vi "humidity_conversions.vi"() -> ()   [LabVIEW 2026]
panel:
  out "RH SIM":dbl
  out "Sim RH":dbl(graph)
  out "T(C) SIM":dbl
  out "Td SIM":dbl
  out "Sim T(C)":dynamicdata(graph)
  out "Sim Td":dynamicdata(graph)
  in  "stop":bool
  in  "TRUE = RH over water\nFALSE = RH over ice":bool
  out "K":dbl
  in  "T (C)":dbl
  out "Td - out":dbl
  in  "RH - inp":dbl
  # "CONVERTS RH & TEMP TO DEW POINT"
  # "CONVERTS TEMP & DEW POINT TO RH"
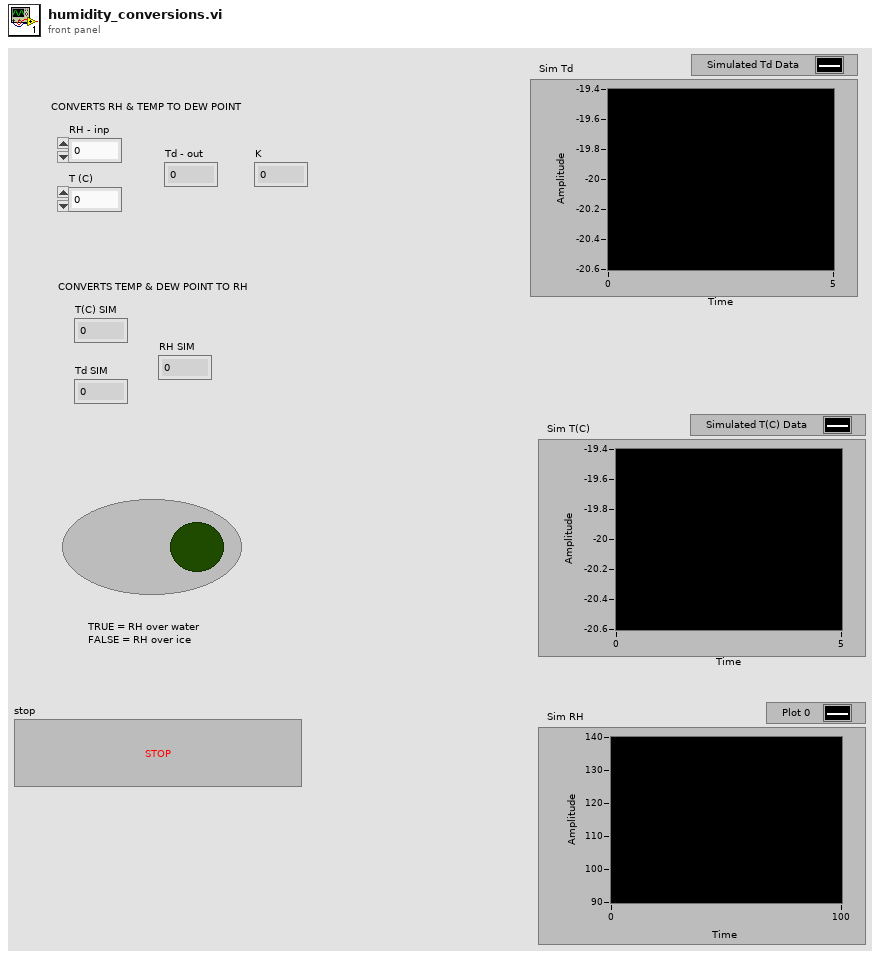
[diagram p1: front panel]
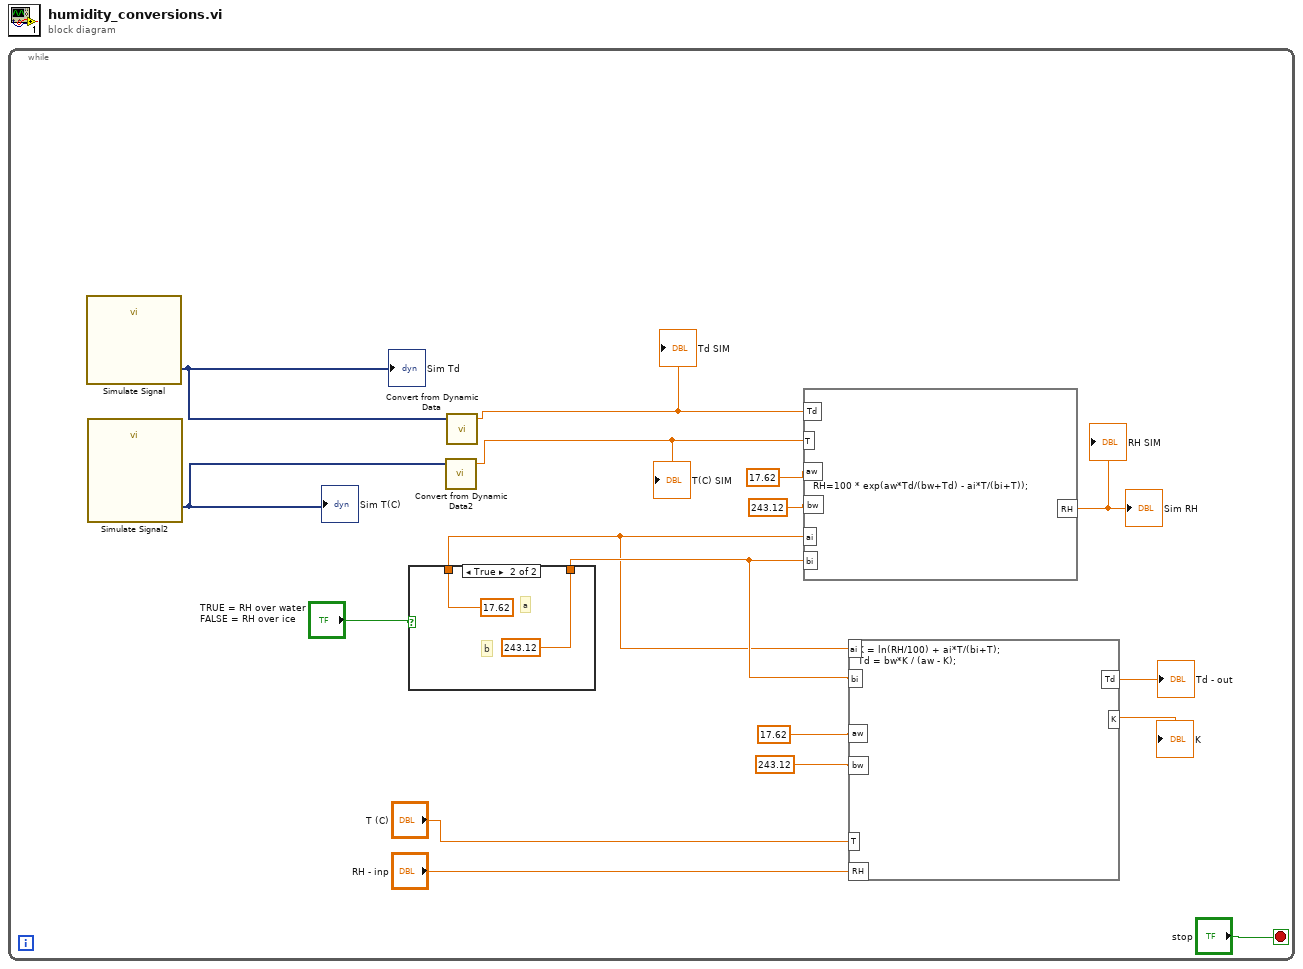
[diagram p0: block diagram]
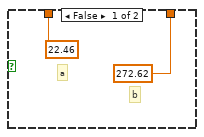
[diagram p2: hidden frame]
diagram:
  n1 = while {
    stop <- "stop" stop-if-true
    n2 = call "Simulate Signal"() -> ("Simulated Td Data"=w5:dynamicdata)  [unwired: 14 in, 1 out]
    "Sim Td" <- w5
    n3 = call "Simulate Signal2"() -> ("Simulated T(C) Data"=w3:dynamicdata)  [unwired: 14 in, 1 out]
    "Sim T(C)" <- w3
    n4 = case shown="True" "TRUE = RH over water\nFALSE = RH over ice" {
      tunnel: [22.46 ("input variable") 17.62 ("input variable")] -> w11
      tunnel: [272.62 ("input variable") 243.12 ("input variable")] -> w14
      frame False {
        # "b"
        # "a"
      }
      frame True {
        # "b"
        # "a"
      }
    }
    n5 = call "Convert from Dynamic Data2"("Dynamic Data Type"=w3) -> ("Scalar"=w2:dbl)  [unwired: 3 in]
    "T(C) SIM" <- w2
    n6 = call "Convert from Dynamic Data"("Dynamic Data Type"=w5) -> ("Scalar"=w4:dbl)  [unwired: 3 in]
    "Td SIM" <- w4
    n7 = formula code="RH=100 * exp(aw*Td/(bw+Td) - ai*T/(bi+T));"("Td"=w4, "T"=w2, "ai"=w11, "bi"=w14, "aw"=17.62 ("input variable"), "bw"=243.12 ("input variable")) -> ("RH"=→"Sim RH" →"RH SIM":dbl)
    n8 = formula code="K = ln(RH/100) + ai*T/(bi+T);\nTd = bw*K / (aw - K);"("RH"="RH - inp", "ai"=w11, "bi"=w14, "T"="T (C)", "aw"=17.62 ("input variable"), "bw"=243.12 ("input variable")) -> ("Td"=→"Td - out":dbl, "K"=→"K":dbl)
  }
